vi "Input.vi"(9 "theta":dbl, 10 "x":dbl, 11 "setpoint":dbl) -> (0 "thetadot_e":dbl, 1 "theta_e":dbl, 2 "xdot_e":dbl, 3 "x_e":dbl)   [LabVIEW 2013]
uses:
  <vilib>/Simulation/Implementation/Shared/SIMSCR Execution Mode.ctl
  <vilib>/Simulation/Scripting/Companion Diagram/SimConfigNode/SimParams.ctl
  <vilib>/Simulation/Scripting/Companion Diagram/SimConfigNode/_simSolvers.ctl
  <vilib>/Simulation/Param Hierarchy/Typedefs/SIMPH Param Control Actions.ctl
  <vilib>/Simulation/Implementation/Shared/NILVSim_ParamChanged.vi
  <vilib>/Simulation/Implementation/Shared/NILVSIM_BeginStep.vi
  <vilib>/Simulation/ContinuousLinear/Implementation/NILVSim Derivative.llb/SIM derivative (scalar).vi
  <vilib>/Simulation/Implementation/Shared/NILVSim_Manager.vi
  <vilib>/Simulation/Implementation/Shared/NILVSim_FinalizeModel.vi
  <vilib>/Simulation/Implementation/Shared/SIM Unbundle Sim Info.vi
  <vilib>/Utility/error.llb/Clear Errors.vi
  <vilib>/Simulation/Implementation/Shared/NILVSim_GetModelError.vi
  <vilib>/Simulation/Implementation/Shared/SIM SimErrorHandler.vi
  <vilib>/Simulation/Implementation/Shared/SIM Bundle Sim Info.vi
  <vilib>/Simulation/Implementation/Shared/SIMSH Read Queue.vi
  <vilib>/Simulation/Implementation/Shared/NILVSim_Initialize.vi
  <vilib>/addons/control/pid/pid.llb/PID Control Input Filter (DBL).vi
  <vilib>/Simulation/Utility/Implementation/NILVSim Get Time and IsAcceptedStep.vi
  <vilib>/Simulation/Scripting/Companion Diagram/SimConfigNode/SimDog.xnode
  <vilib>/Simulation/Implementation/XNodeFramework/SimXNode/SimX.xnode
  <vilib>/addons/control/pid/NI_PID_pid.lvlib
  <vilib>/Simulation/Implementation/Shared/NI_SIM_Implementation.lvlib
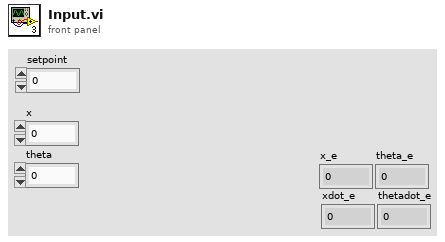
[diagram p1: front panel]
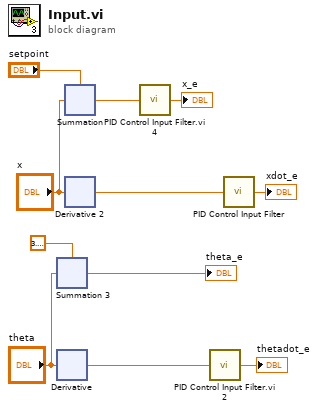
[diagram p0: block diagram]
diagram:
  n1 = xnode "Summation 3"("Operand1"=3.141592653589793 ("Constant"), "Operand2"="theta") -> ("Result"=→"theta_e":dbl)
  n2 = xnode "Derivative"("input"="theta") -> ("output"=w3:dbl)  [unwired: 2 in]
  n3 = xnode "Summation"("Operand1"="setpoint", "Operand2"="x") -> ("Result"=w6:dbl)
  n4 = xnode "Derivative 2"("input"="x") -> ("output"=w2:dbl)  [unwired: 2 in]
  n5 = call-poly "PID Control Input Filter.vi 4"("input"=w6) -> ("output"=→"x_e":dbl)  [unwired: 4 in]
  n6 = call-poly "PID Control Input Filter.vi 2"("input"=w3) -> ("output"=→"thetadot_e":dbl)  [unwired: 4 in]
  n7 = call-poly <vilib>:"PID Control Input Filter.vi"("input"=w2) -> ("output"=→"xdot_e":dbl)  [unwired: 4 in]
